vi "Select Goal Position.vi"(8 "Distance Limit (pixels)":sgl=2.0, 10 "Goal In":cluster{"X Centroid":sgl, "Y Centroid":sgl}, 11 "Goal Previous":cluster{"X Centroid":sgl, "Y Centroid":sgl}) -> (3 "Goal Out":cluster{"X Centroid":sgl, "Y Centroid":sgl} {"Y Centroid" format="%.2f"; "X Centroid" format="%.2f"})   [LabVIEW 2012]
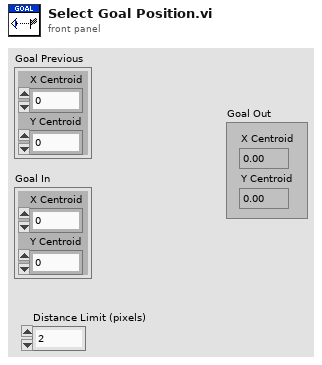
[diagram p1: front panel]
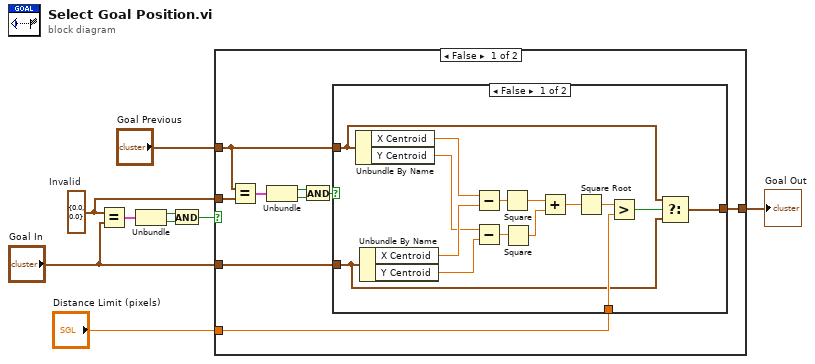
[diagram p0: block diagram]
diagram:
  w2 = cluster{"X Centroid":sgl, "Y Centroid":sgl} {"X Centroid"=0.0, "Y Centroid"=0.0}  # Invalid
  n1 = Equal?(x=w2, y="Goal In") -> (x = y?=w7:cluster{"X Centroid":bool, "Y Centroid":bool})
  n2 = Unbundle(w7) -> ("X Centroid"=w6:bool, "Y Centroid"=w5:bool)
  n3 = And(x=w6, y=w5) -> (x .and. y?=w4:bool)
  n4 = case shown="False" w4 {
    tunnel: "Goal In" -> [w18 _]
    tunnel: "Goal Previous" -> [w13 w35]
    tunnel: [w11 w35] -> w3
    tunnel: w2 -> [w12 _]
    tunnel: "Distance Limit (pixels)" -> [w10 _]
    frame False {
      n5 = Equal?(x=w13, y=w12) -> (x = y?=w15:cluster{"X Centroid":bool, "Y Centroid":bool})
      n6 = Unbundle(w15) -> ("X Centroid"=w16:bool, "Y Centroid"=w17:bool)
      n7 = And(x=w16, y=w17) -> (x .and. y?=w14:bool)
      n8 = case shown="False" w14 {
        tunnel: w18 -> [w20 w34]
        tunnel: w13 -> [w21 _]
        tunnel: [w19 w34] -> w11
        tunnel: w10 -> [w23 _]
        frame False {
          n9 = Unbundle By Name(w21) -> ("X Centroid"=w33:sgl, "Y Centroid"=w31:sgl)
          n10 = Unbundle By Name(w20) -> ("X Centroid"=w32:sgl, "Y Centroid"=w30:sgl)
          n11 = Subtract(x=w33, y=w32) -> (x-y=w29:sgl)
          n12 = Subtract(x=w31, y=w30) -> (x-y=w28:sgl)
          n13 = Square(x=w29) -> (x^2=w26:sgl)
          n14 = Square(x=w28) -> (x^2=w27:sgl)
          n15 = Add(x=w26, y=w27) -> (x+y=w25:sgl)
          n16 = Square Root(x=w25) -> (sqrt(x)=w24:sgl)
          n17 = Greater?(x=w24, y=w23) -> (0:w22:bool)
          n18 = Select(t=w21, s=w22, f=w20) -> (s? t:f=w19:cluster{"X Centroid":sgl, "Y Centroid":sgl})
        }
        frame True {
        }
      }
    }
    frame True {
    }
  }
  "Goal Out" <- w3
